vi "Configure Trigger Mode.vi"(8 "error in (no error)":errorcluster, 10 "trigger mode (Single)":T1 items=["Single", "Continuous", "Gated", "Burst"], 11 "VISA resource name":refnum<visa-resource-name>) -> (0 "error out":errorcluster, 3 "VISA resource name out":refnum<visa-resource-name>)   [LabVIEW 2019, in "Pulse Rider PG-1000.lvlib"]
doc: "Set the instrument trigger source.\nThe trigger mode can be : gated, single, burst, continuous"
uses:
  <instrlib>/Pulse Rider PG-1000/Pulse Rider PG-1000.lvlib
  <instrlib>/Pulse Rider PG-1000/Public/Configure/Trigger/Trigger Mode.ctl
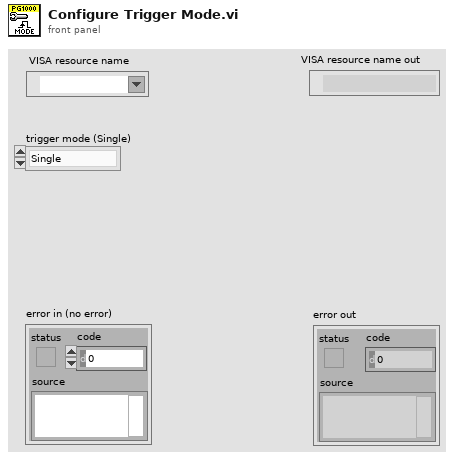
[diagram p1: front panel]
types:
  T1 = typedef "Pulse Rider PG-1000.lvlib/Trigger Mode.ctl" = u16
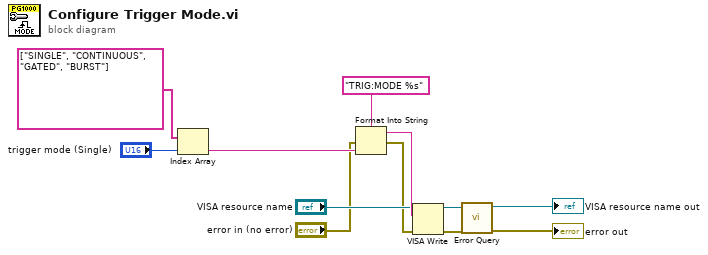
[diagram p0: block diagram]
diagram:
  n1 = Index Array(array=string[] ["SINGLE", "CONTINUOUS", "GATED", "BURST"], index="trigger mode (Single)") -> (element=w3:string)
  n2 = Format Into String(format string="TRIG:MODE %s", error in="error in (no error)", w3) -> (resulting string=w9:string, error out=w1:errorcluster)  [unwired: 1 in]
  n3 = VISA Write(VISA resource name="VISA resource name", write buffer=w9, error in (no error)=w1) -> (VISA resource name out=w12:refnum<visa-resource-name>, error out=w11:errorcluster)  [unwired: 1 out]
  n4 = call <instrlib>:"Error Query.vi"("error in (no error)"=w11, "VISA resource name"=w12) -> ("error out"=→"error out":errorcluster, "VISA resource name out"=→"VISA resource name out":refnum<visa-resource-name>)  [unwired: 6 in, 2 out]
